vi "Set settings chain.vi"(8 "error in (no error)":errorcluster, 9 "class name":string[](array[string]), 10 "settings":variant[](array[variant]), 11 "ExampleClassA in":refnum<class "ExampleClassA.lvclass">) -> (0 "error out":errorcluster, 3 "ExampleClassA out":refnum<class "ExampleClassA.lvclass">)   [LabVIEW 2012, in "ExampleClassA.lvclass"]
uses:
  ExampleClassA.lvclass
  <vilib>/Distrio/Murmex/Murmex/Murmex.lvclass
  ExampleClassA.lvclass/ExampleClassA.ctl
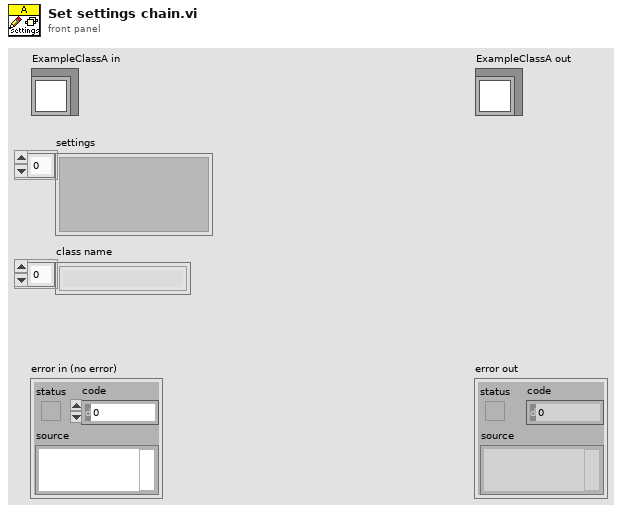
[diagram p1: front panel]
types:
  T1 = typedef "ExampleClassA.lvclass/Settings cluster.ctl" = cluster{"period?":dbl[unit], "number of blocks":i32, "number of channels":i32}
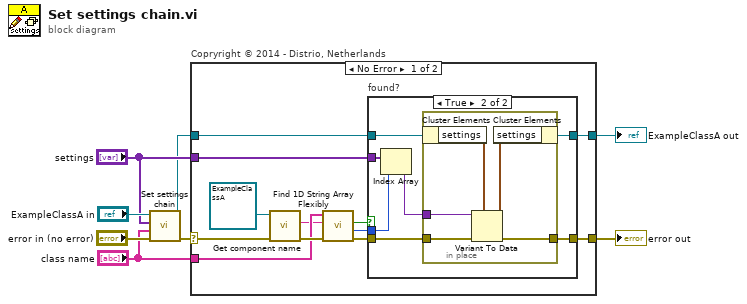
[diagram p0: block diagram]
diagram:
  n1 = call-parent "Set settings chain.vi"("error in (no error)"="error in (no error)", "class names"="class name", "settings"="settings", "Murmex in"="ExampleClassA in") -> ("error out"=w5:errorcluster, "Murmex out"=w1:refnum<class "ExampleClassA.lvclass">)  [unwired: 6 in]
  n2 = case "Copryright © 2014 - Distrio, Netherlands" shown="No Error" w5 {
    selector: w5 -> [w20 w36]
    tunnel: [w17 w36] -> w3
    tunnel: [w18 w35] -> w2
    tunnel: "class name" -> [w14 _]
    tunnel: "settings" -> [w19 _]
    tunnel: w1 -> [w10 w35]
    frame No Error {
      n3 = call <vilib>:"Get component name.vi"("error in (no error)"=w20, "Murmex in"=refnum<class "ExampleClassA.lvclass"> refnum ("ExampleClassA in")) -> ("error out"=w16:errorcluster, "component name"=w13:string)  [unwired: 7 in, 1 out]
      n4 = call <vilib>:"Find 1D String Array Flexibly.vi"("error in (no error)"=w16, "element"=w13, "array"=w14) -> ("error out"=w15:errorcluster, "index of element"=w12:i32, "found?"=w11:bool)  [unwired: 6 in]
      n5 = case "found?" shown="True" w11 {
        tunnel: w19 -> [_ w29]
        tunnel: w10 -> [w22 w27]
        tunnel: [w22 w26] -> w18
        tunnel: [w21 w25] -> w17
        tunnel: w15 -> [w21 w24]
        tunnel: w12 -> [_ w23]
        frame False {
        }
        frame True {
          n6 = Index Array(array=w29, index=w23) -> (element=w28:variant)
          n7 = in-place {
            in-place-border: w28 -> [w34]
            in-place-border: w24 -> [w32]
            in-place-border: [w30] -> w25
            n8 = in-place-cluster #1(w27) -> ("settings"=w33:T1)
            n9 = Variant To Data(error in=w32, type=w33, Variant=w34) -> (data=w31:T1, error out=w30:errorcluster)
            n10 = in-place-cluster #1("settings"=w31) -> (w26:refnum<class "ExampleClassA.lvclass">)
          }
        }
      }
    }
    frame Error {
    }
  }
  "error out" <- w3
  "ExampleClassA out" <- w2
